vi "XML ( Clone and Append Single Input ).vi"(8 "error in (no error)":errorcluster, 9 "Parent_Node":string, 10 "Clone_Node":string, 11 "XML in":refnum<class "XML.lvclass">) -> (0 "error out":errorcluster, 3 "XML out":refnum<class "XML.lvclass">)   [LabVIEW 2018, in "XML.lvlib" / "XML.lvclass"]
uses:
  XML.lvclass
  XML.lvclass/XML.ctl
  <vilib>/xml/Close Reference(Node).vi
  <vilib>/xml/NI_XML.lvlib
  <resource>/objmgr/DOMUserDefRef.rc
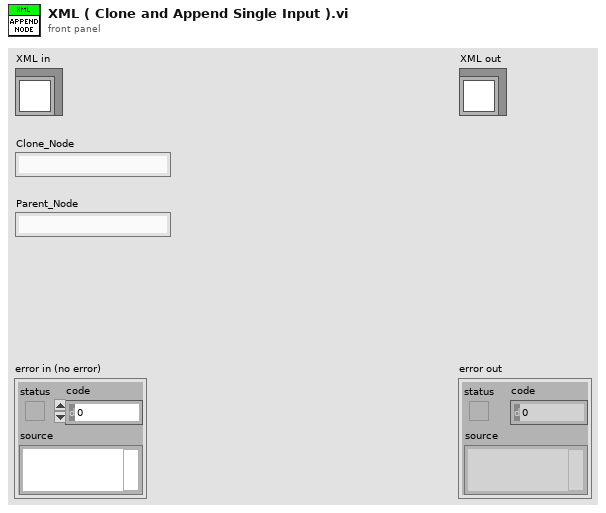
[diagram p1: front panel]
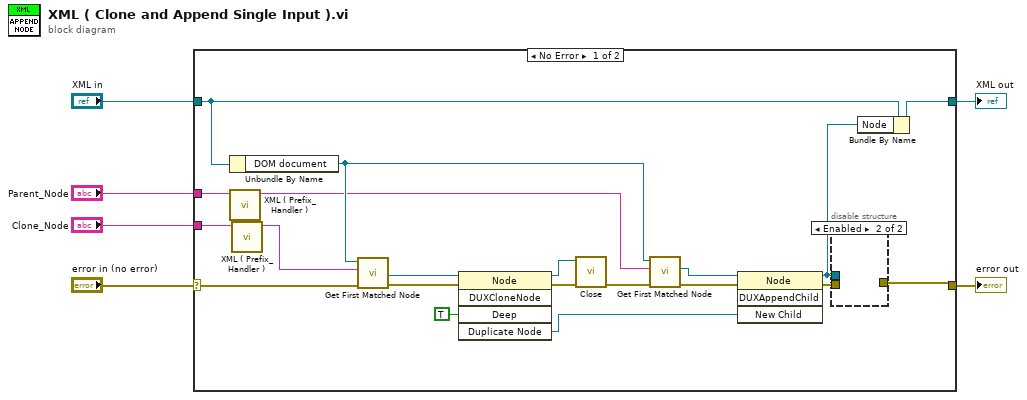
[diagram p0: block diagram]
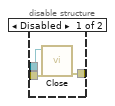
[diagram p2: hidden frame]
diagram:
  n1 = case shown="No Error" "error in (no error)" {
    selector: "error in (no error)" -> [w21 w31]
    tunnel: [w14 w31] -> w5
    tunnel: [w9 w30] -> w3
    tunnel: "XML in" -> [w26 w30]
    tunnel: "Clone_Node" -> [w25 _]
    tunnel: "Parent_Node" -> [w12 _]
    frame No Error {
      n2 = Unbundle By Name(w26) -> ("DOM document"=w13:refnum<k20>)
      n3 = call "XML ( Prefix_Handler ).vi"("input string"=w12) -> ("result string"=w11:string)  [unwired: 10 in]
      n4 = call "XML ( Prefix_Handler ).vi"("input string"=w25) -> ("result string"=w10:string)  [unwired: 10 in]
      n5 = call <vilib>:"Get First Matched Node.vi"("error in (no error)"=w21, "XPath expression"=w10, "node in"=w13) -> ("error out"=w20:errorcluster, "node result"=w24:refnum<k20>)  [unwired: 6 in, 1 out]
      n6 = invoke class="Node" method="DUXCloneNode"(reference=w24, error in=w20, "Deep"=TRUE) -> (reference out=w18:refnum<k20>, error out=w19:errorcluster, "Duplicate Node"=w8:refnum<k20>)  [unwired: 2 in, 2 out]
      n7 = call-poly <vilib>:"Close.vi"("error in (no error)"=w19, "node"=w18) -> ("error out"=w16:errorcluster)  [unwired: 7 in]
      n8 = call <vilib>:"Get First Matched Node.vi"("error in (no error)"=w16, "XPath expression"=w11, "node in"=w13) -> ("error out"=w22:errorcluster, "node result"=w17:refnum<k20>)  [unwired: 6 in, 1 out]
      n9 = invoke class="Node" method="DUXAppendChild"(reference=w17, error in=w22, "New Child"=w8) -> (reference out=w7:refnum<k20>, error out=w15:errorcluster)  [unwired: 1 in, 2 out]
      n10 = disable-structure shown="Enabled" {
        disable-tunnel: w15 -> [w29 _]
        disable-tunnel: w7 -> [w28 _]
        disable-tunnel: [w27 _] -> w14
        frame Disabled {
          n11 = call-poly <vilib>:"Close.vi"("error in (no error)"=w29, "node"=w28) -> ("error out"=w27:errorcluster)  [unwired: 7 in]
        }
        frame Enabled {
        }
      }
      n12 = Bundle By Name(cluster=w26, "Node"=w7) -> (w9:refnum<class "XML.lvclass">)
    }
    frame Error {
    }
  }
  "error out" <- w5
  "XML out" <- w3
